vi "main.vi"() -> ()   [LabVIEW 2020]
uses:
  Controls/UI_Cluster.ctl
panel:
  out "I całkujacy":dbl
  out "e uchyb":dbl
  out "c [%] z regulatora":dbl
  in  "Twy [°C] zadane":dbl
  out "Regulator PI":bool
  in  "Dt [s]":dbl=0.2 min=0.2 max=5.0 step=0.1
  out "Wszystko manualnie":bool
  out "Dane wejściowe z pliku":bool
  out "c [%] Moc grzałki z pliku":dbl
  out "Twe [°C] z pliku":dbl
  out "F [L/min] z pliku":dbl
  in  "Radio Buttons":T1(radio)
  in  "Cancel Button":bool
  out "String":string
  in  "Start":bool
  out "Wykres Twy":dbl(graph)
  in  "V [L]":dbl min=0.0
  in  "Prędkość symulacji x":u32(slide) scale=1.0..100.0
  out "Twy [°C]":dbl
  in  "c [%]":dbl min=0.0 max=100.0
  in  "F [L/min]":dbl=5.0 min=0.0
  in  "Twe [°C]":dbl=30.0
  in  "stop":bool
  # "--------------------Dane podane manulanie---------------------"
  # "-----------Dane z pliku-----------"
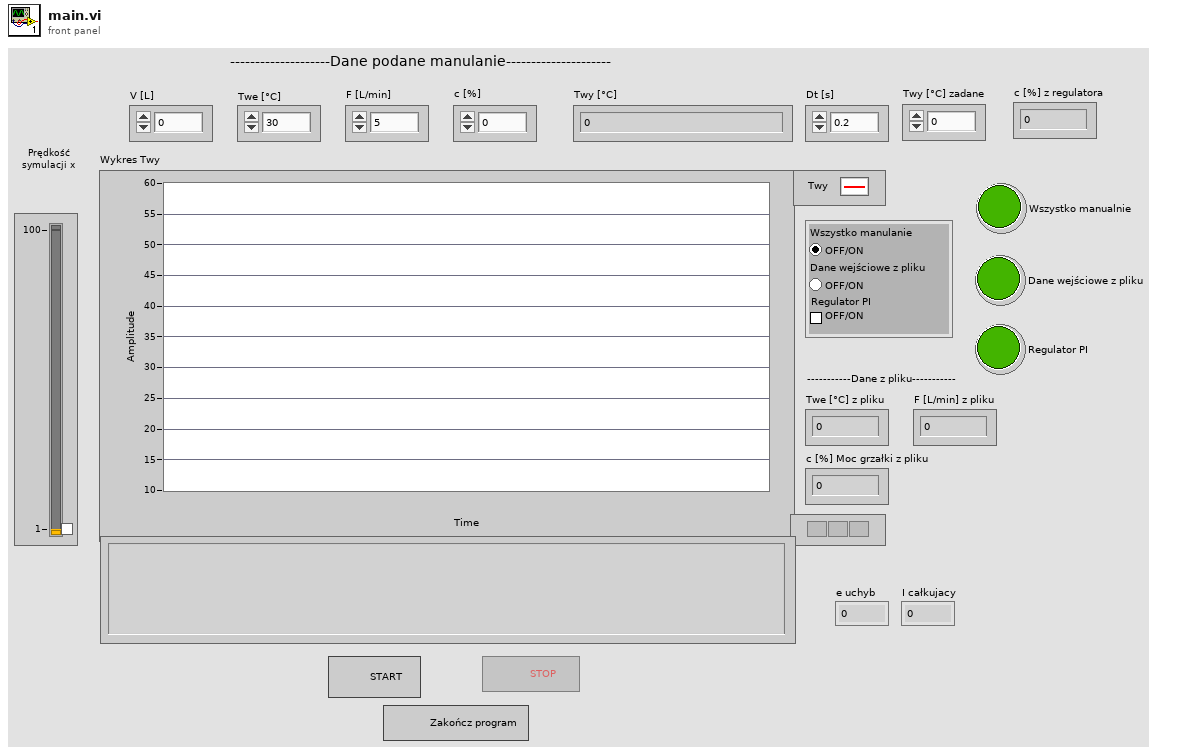
[diagram p1: front panel]
types:
  T1 = enum32{"Wszystko manulanie", "Dane wejściowe z pliku", "Regulator PI"}
  T2 = enum32{"Invalid", "Standard", "Closed", "Hidden", "Minimized", "Maximized"}
  T3 = enum32{"invalid app kind", "Development System", "Run Time System", "Student Edition", "Embedded LabVIEW", "Evaluation", "Custom"}
  T4 = enum16{"open", "replace", "create", "open or create", "replace or create", "replace or create with confirmation"}
  T5 = typedef "UI_Cluster.ctl" = cluster{"krok całkowania Ref":refnum<vi>, "c [%] Ref":refnum<vi>, "F [L/min] Ref":refnum<vi>, "V [L] Ref":refnum<vi>, "Twe Ref":refnum<vi>, "Wykres Twy Ref":refnum<vi>, "String Ref":refnum<vi>, "Start Ref":refnum<vi>, "stop Ref":refnum<vi>, "End Ref":refnum<vi>, "Dane wejściowe z pliku Ref":refnum<vi>, "Wszystko manualnie Ref":refnum<vi>, "Dt Refnum":refnum<vi>, "Radio Buttons Ref":refnum<vi>}
  T6 = cluster{"Core":cluster{"Current VI Reference":refnum<vi>, "Close Panel on Exit?":bool}, "Cluster_OUT":T5}
  T7 = cluster{"Current VI Reference":refnum<vi>, "Close Panel on Exit?":bool}
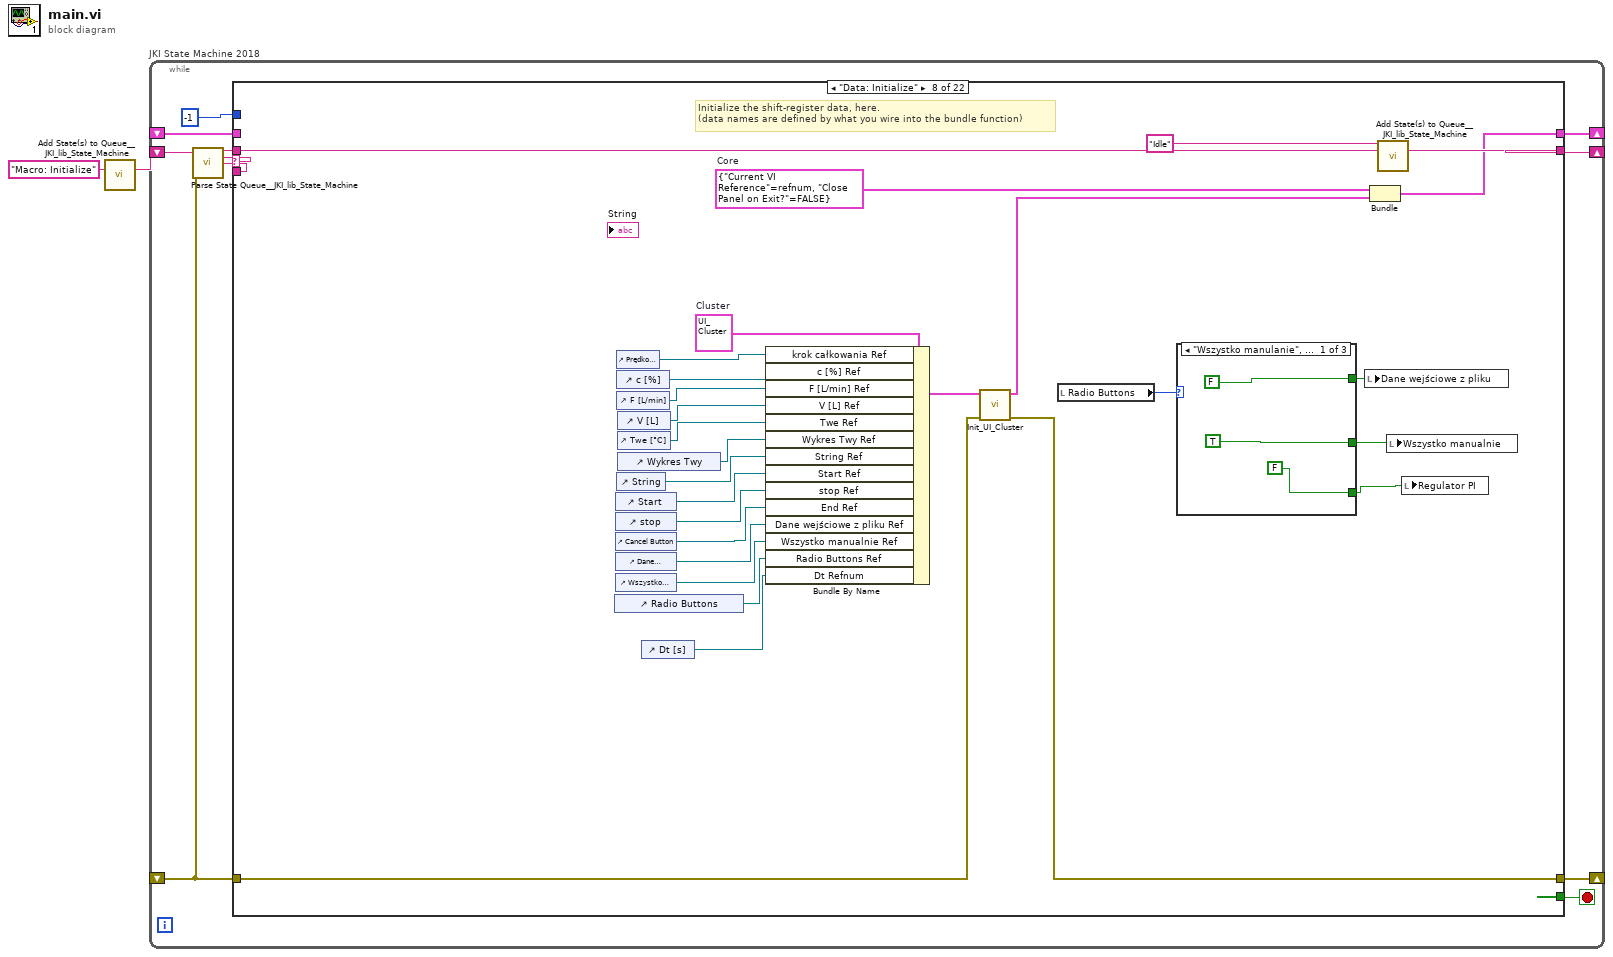
[diagram p0: block diagram]
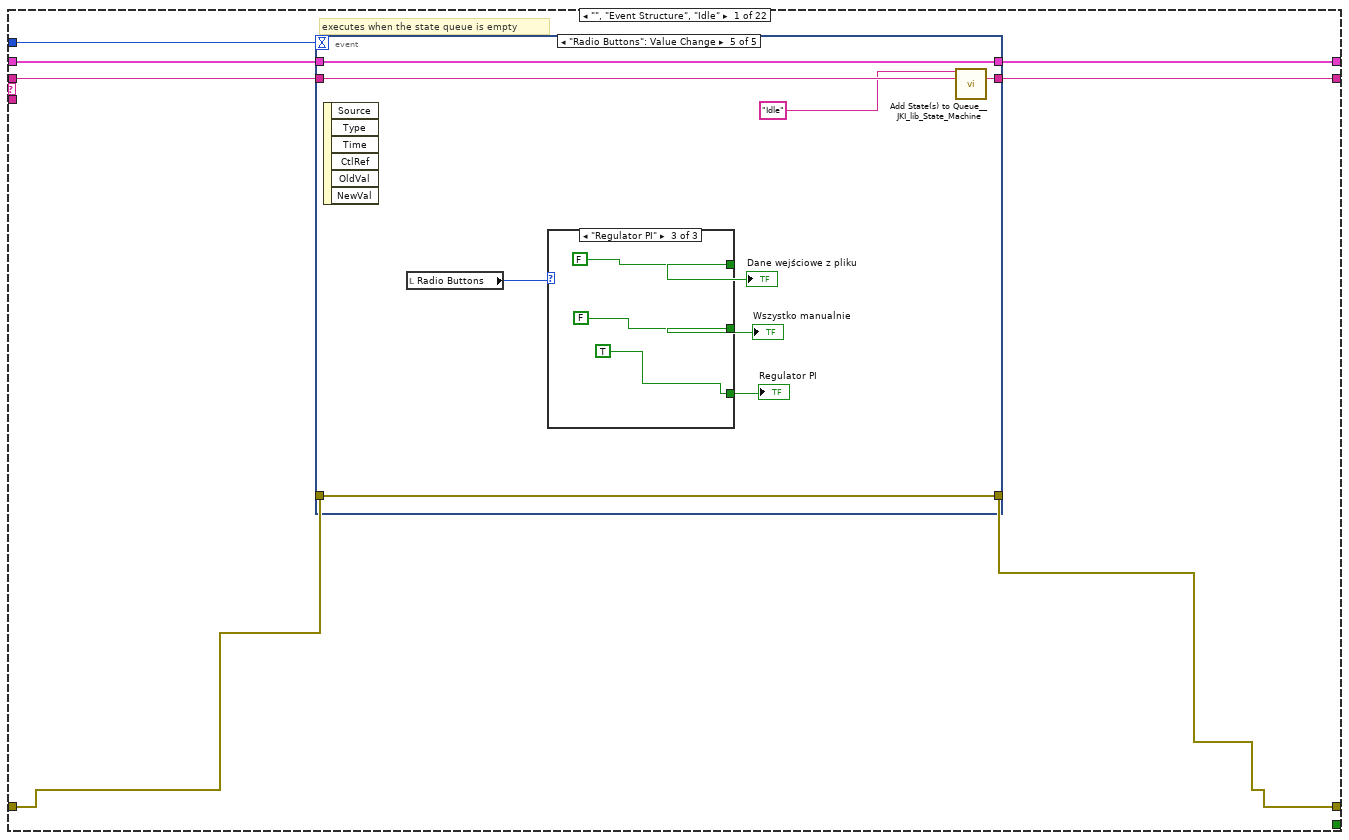
[diagram p2: hidden frame]
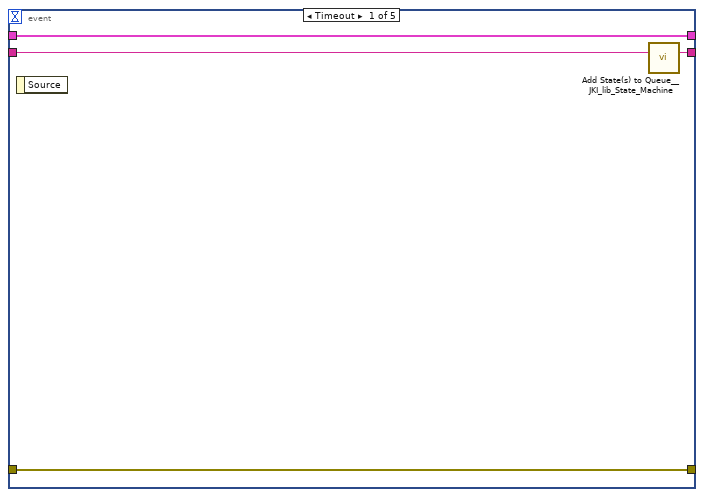
[diagram p3: hidden frame]
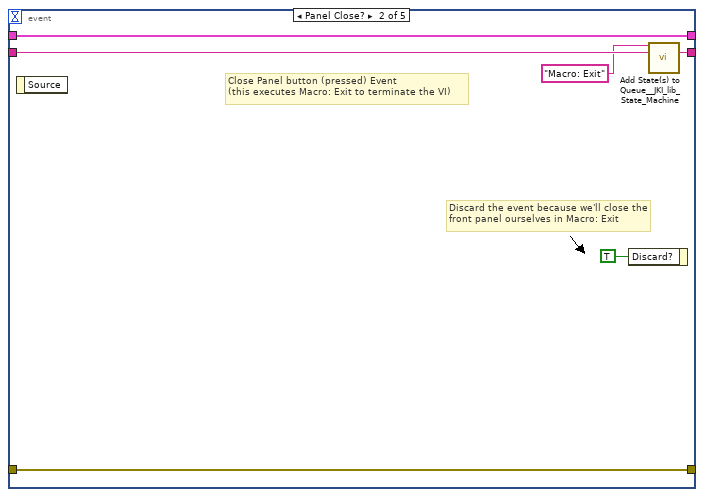
[diagram p4: hidden frame]
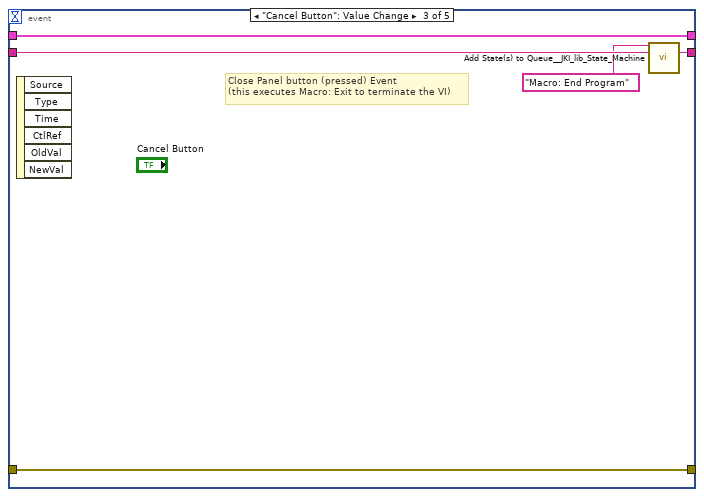
[diagram p5: hidden frame]
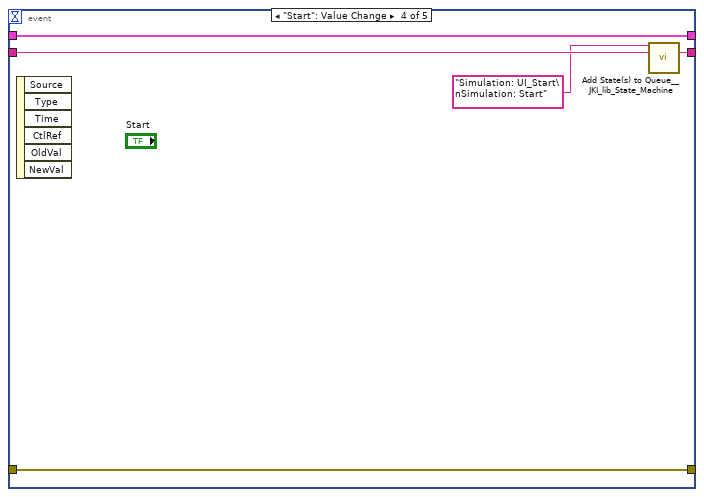
[diagram p6: hidden frame]
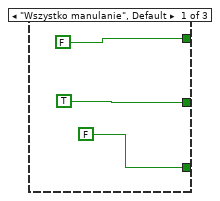
[diagram p7: hidden frame]
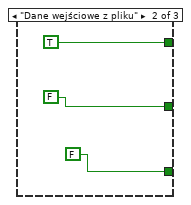
[diagram p8: hidden frame]
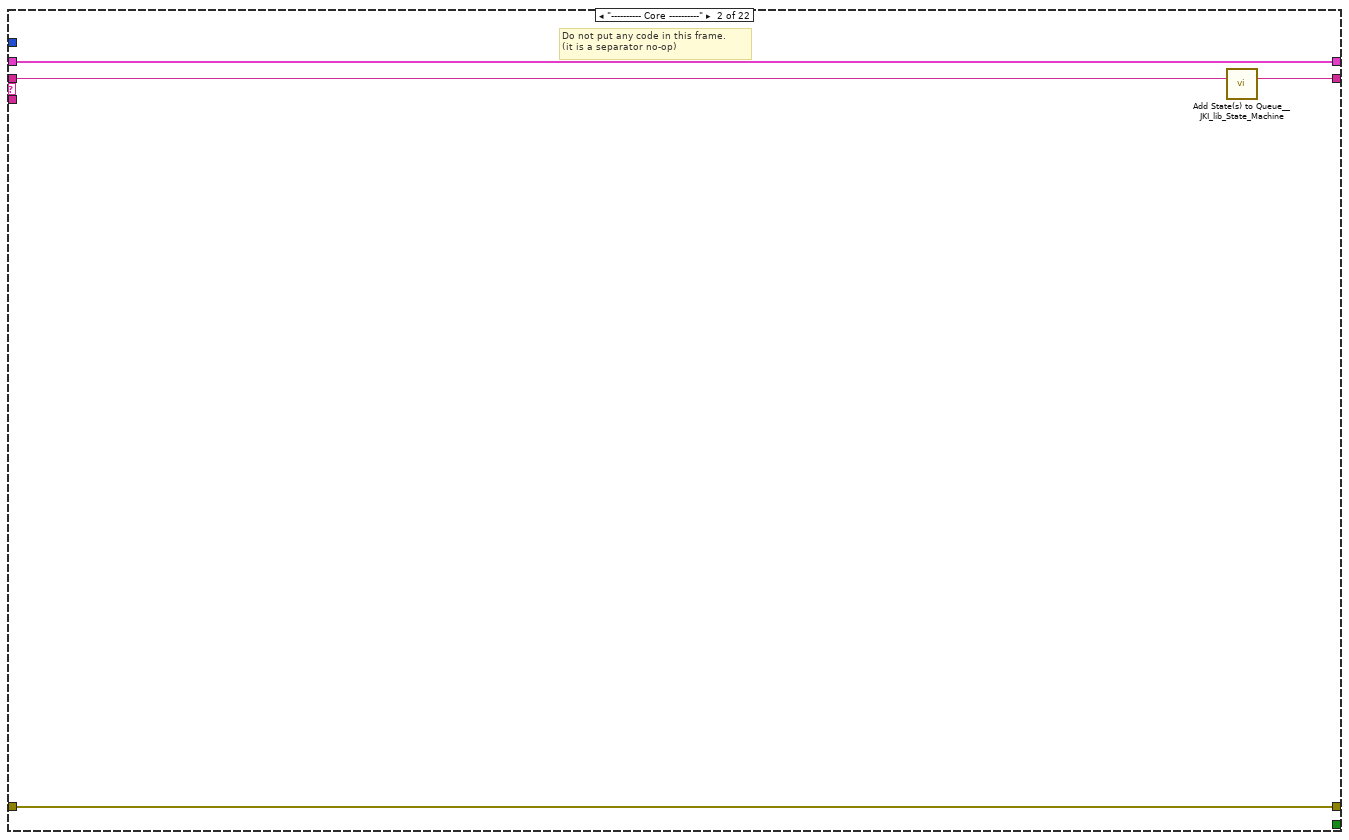
[diagram p9: hidden frame]
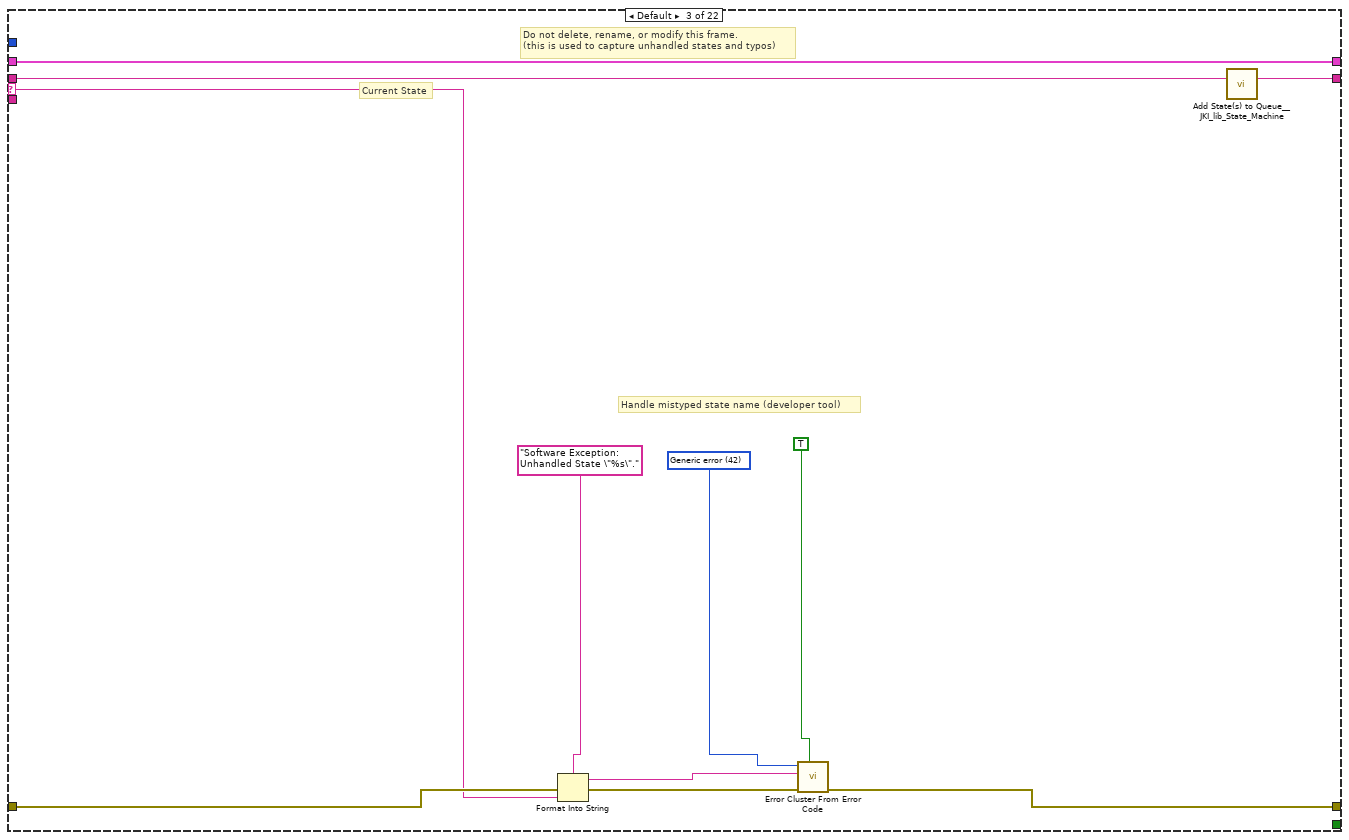
[diagram p10: hidden frame]
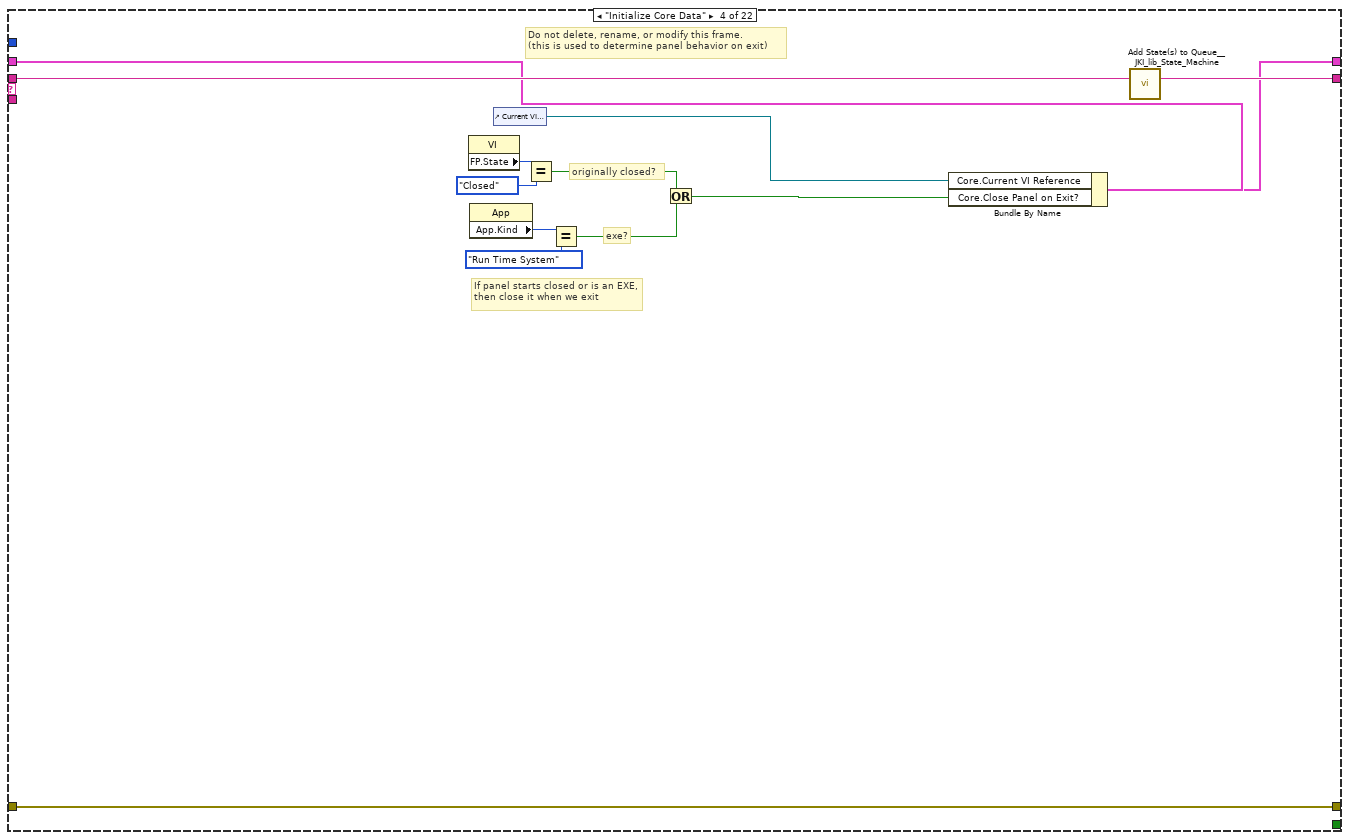
[diagram p11: hidden frame]
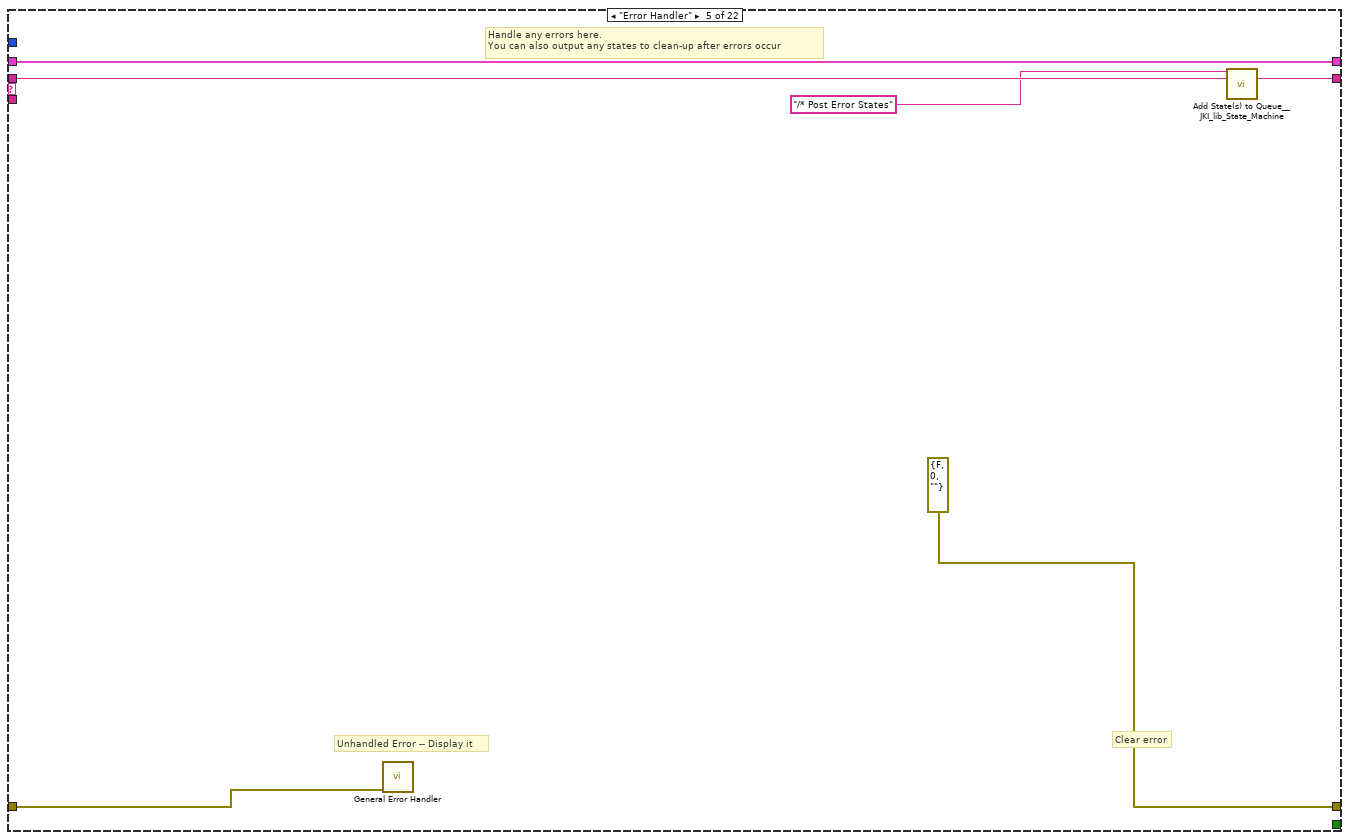
[diagram p12: hidden frame]
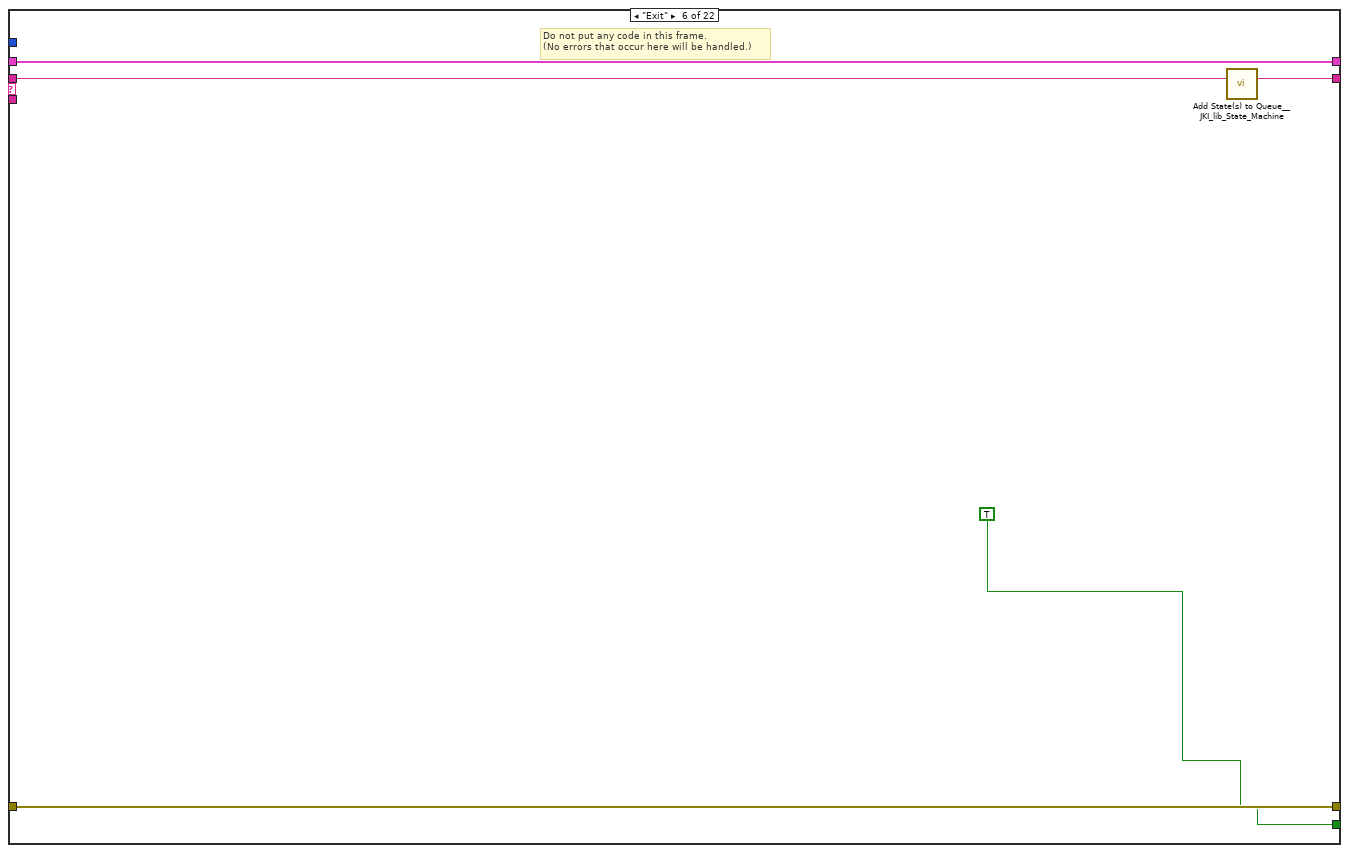
[diagram p13: hidden frame]
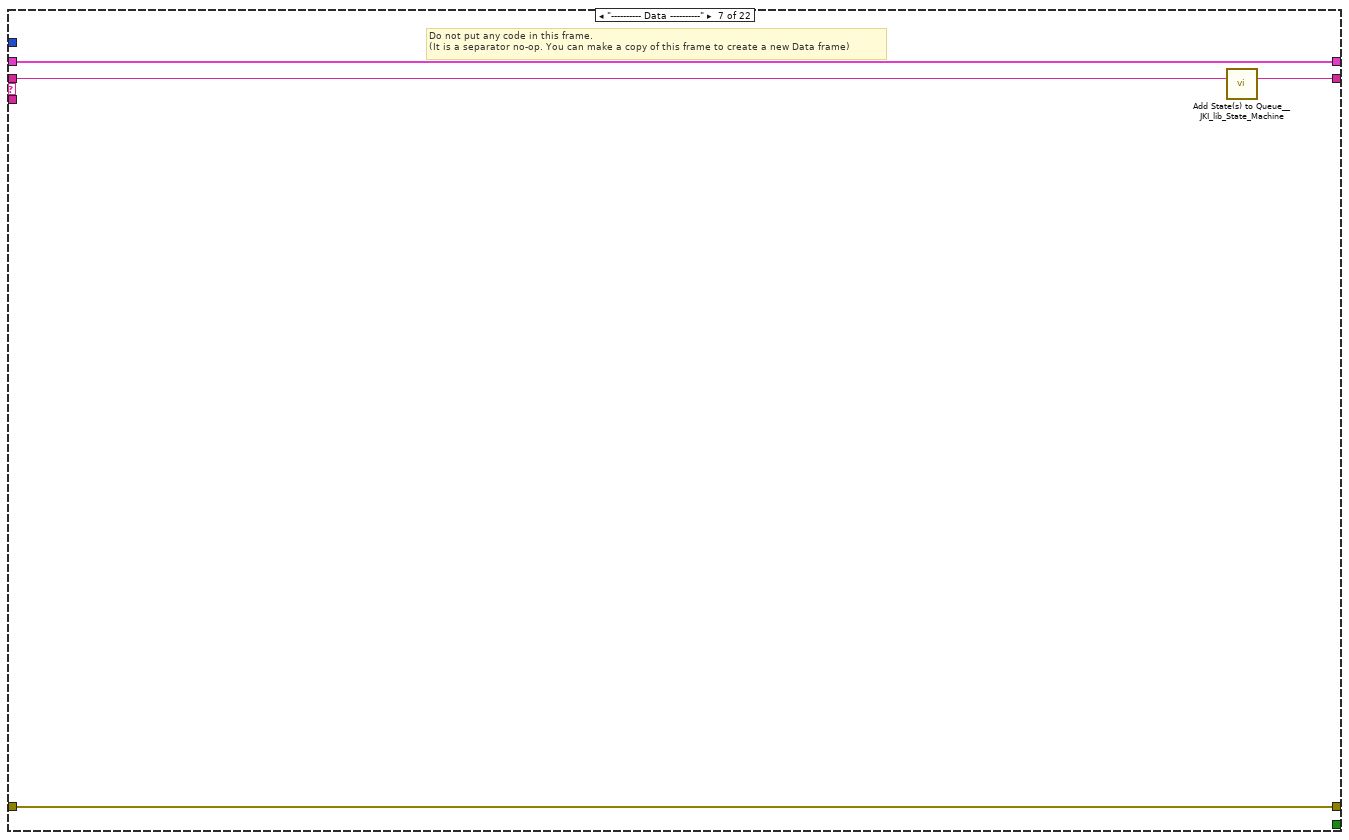
[diagram p14: hidden frame]
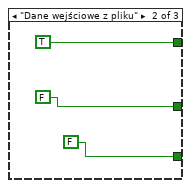
[diagram p15: hidden frame]
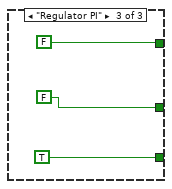
[diagram p16: hidden frame]
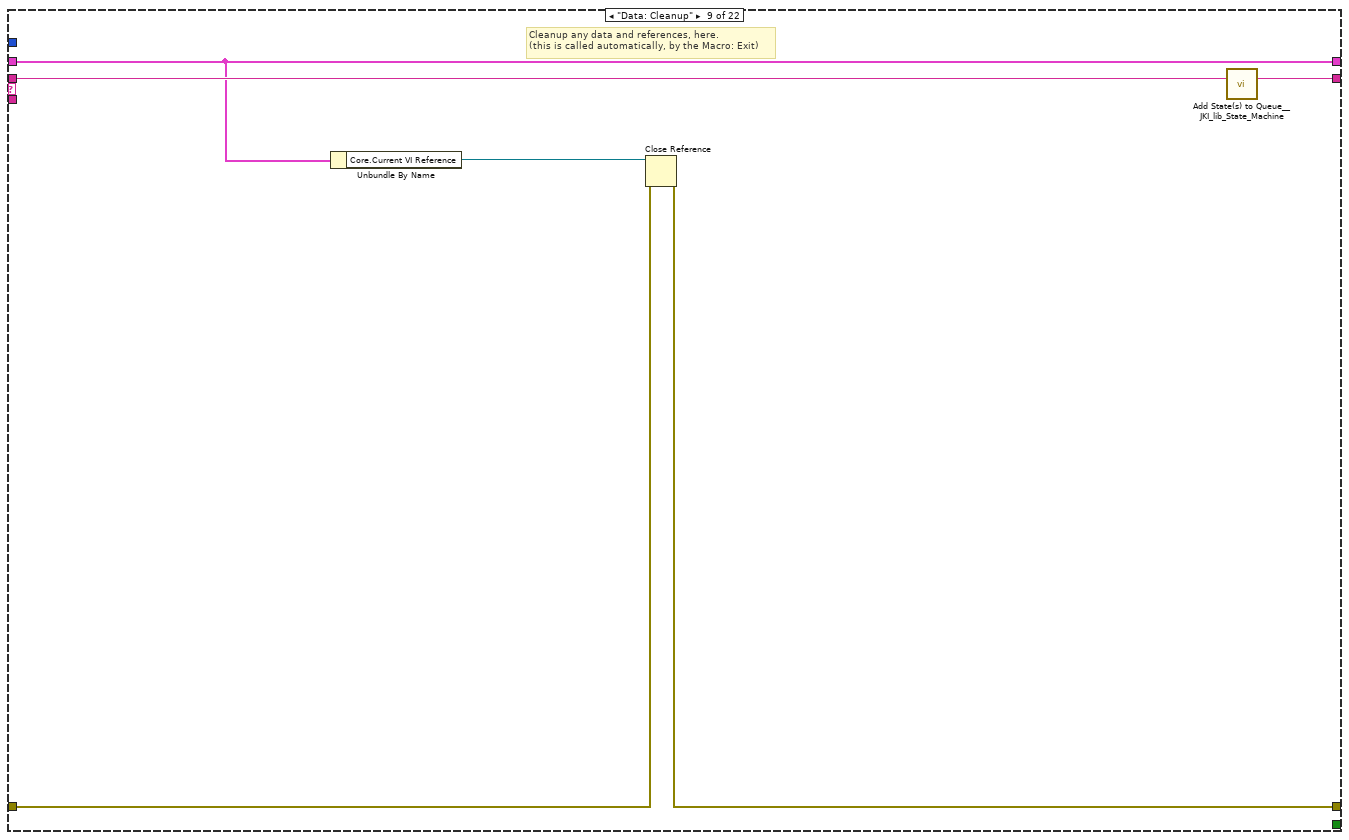
[diagram p17: hidden frame]
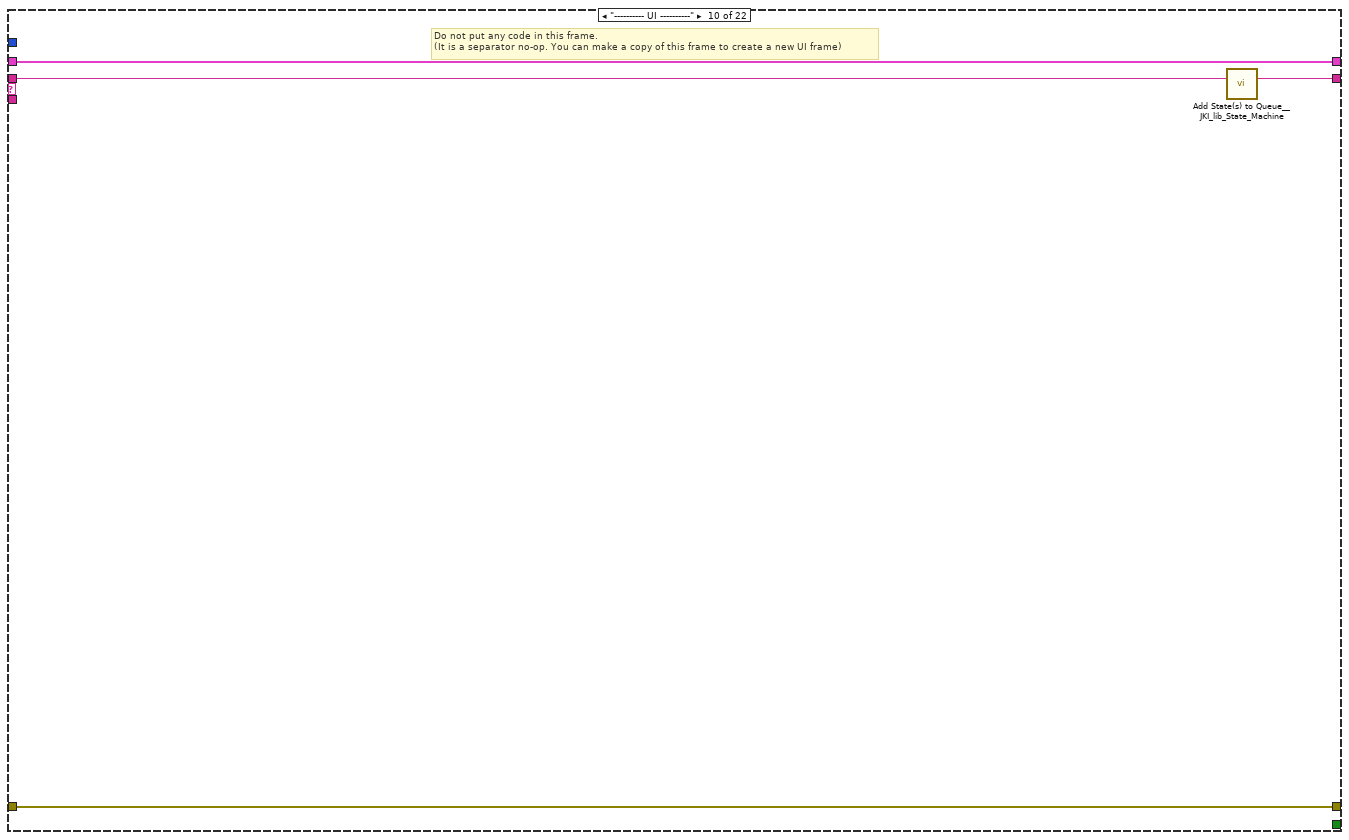
[diagram p18: hidden frame]
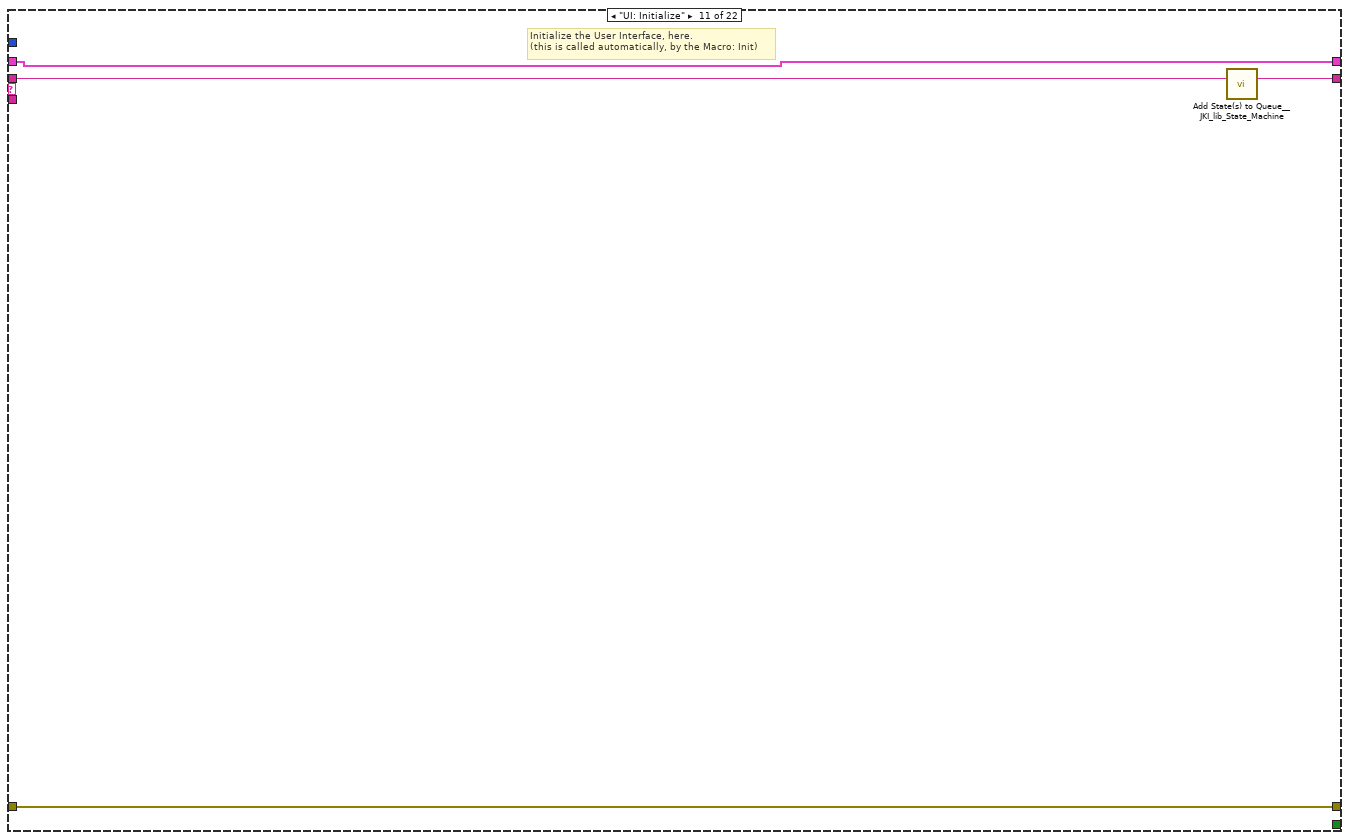
[diagram p19: hidden frame]
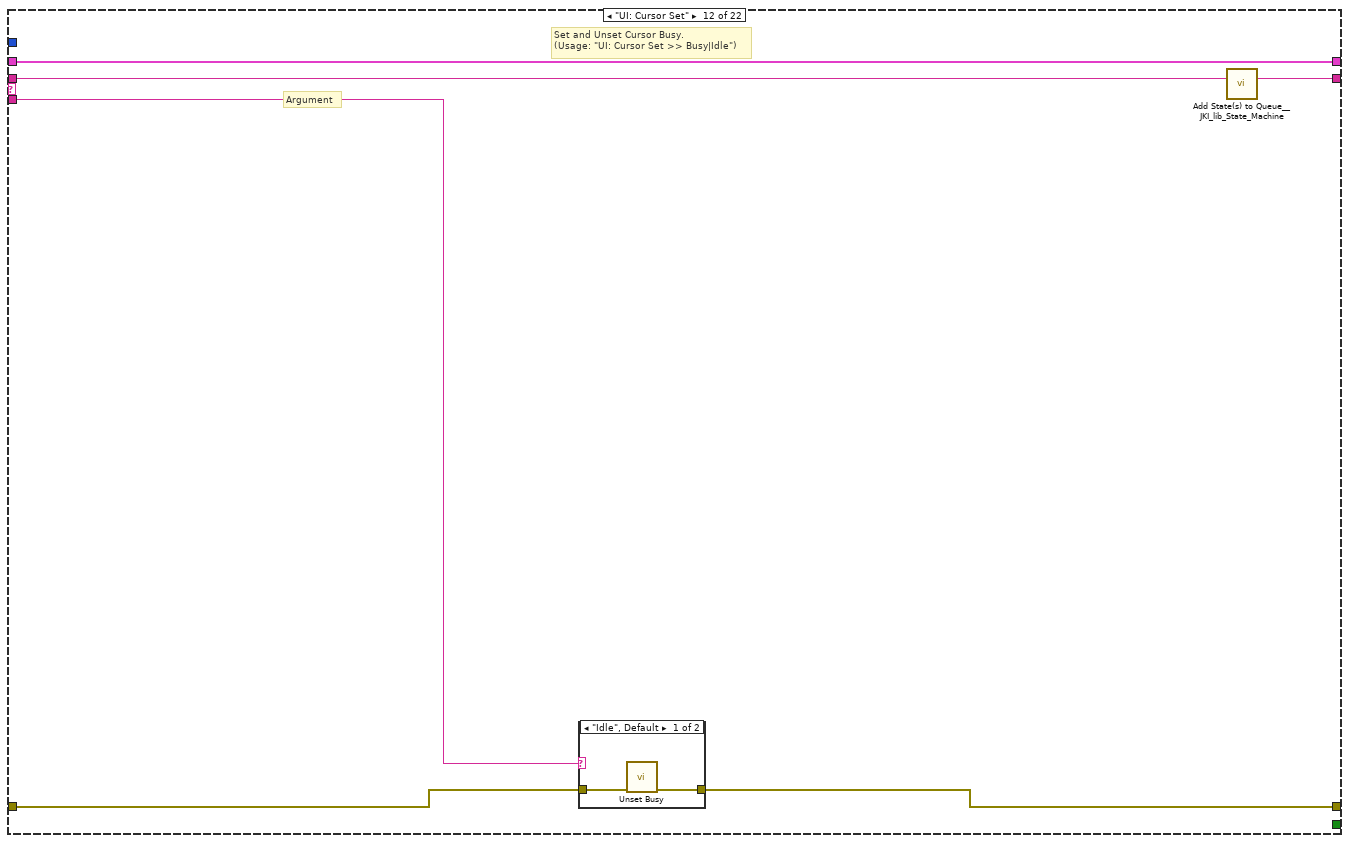
[diagram p20: hidden frame]
diagram:
  n1 = call <vilib>:"Add State(s) to Queue__JKI_lib_State_Machine.vi"("State(s) in (\"\")"="Macro: Initialize") -> ("States Out"=w2:string)  [unwired: 14 in]
  n2 = while "JKI State Machine 2018" {
    shift-right: [w6] -> _
    shift-left: _ -> [w5]
    shift-right: [w9] -> _
    shift-left: _ -> [w3]
    shift-right: [w8] -> _
    shift-left: w2 -> [w10]
    stop <- w7 stop-if-true
    n3 = call <vilib>:"Parse State Queue__JKI_lib_State_Machine.vi"("State Queue"=w10, "Error In (no error)"=w3) -> ("Remaining States"=w12:string, "Current State"=w13:string, "Arguments"=w11:string)  [unwired: 11 in]
    n4 = case shown="\"Data: Initialize\"" w13 {
      selector: w13 -> [_ _ w63 _ _ _ _ _ _ _ _ _ _ _ _ _ _ _ _ _ _ _]
      tunnel: w12 -> [w20 w62 w67 w86 w92 w97 w101 w129 w144 w148 w152 w158 w169 w234 w239 w249 w259 w263 w272 w282 w311 w393]
      tunnel: w11 -> [_ _ _ _ _ _ _ _ _ _ _ w153 w164 _ _ _ _ _ _ _ _ _]
      tunnel: w5 -> [w18 w59 w65 w75 w89 w95 w98 _ w140 w145 w150 w156 w163 w231 w236 w241 w256 w260 w270 w280 w308 w390]
      tunnel: [w17 w60 w69 w84 errorcluster {"status"=FALSE, "code"=0, "source"=""} ("error out") w94 w99 w117 w141 w146 w149 w154 w166 w232 w237 w247 w250 w261 w264 w275 w309 w391] -> w9
      tunnel: w3 -> [w16 w60 w68 w84 w88 w94 w99 w118 w142 w146 w149 w155 w167 w232 w237 w247 w252 w261 w265 w274 w309 w391]
      tunnel: [w19 w61 w66 w85 w91 w96 w100 w128 w143 w147 w151 w157 w168 w233 w238 w248 w258 w262 w271 w281 w310 w392] -> w8
      tunnel: [_ _ _ _ _ TRUE _ _ _ _ _ _ _ _ _ _ TRUE _ _ _ _ _] -> w7
      tunnel: [w15 w59 w65 w74 w89 w95 w98 w115 w140 w145 w150 w156 w163 w231 w236 w241 w256 w260 w266 w278 w308 w390] -> w6
      tunnel: -1 ("Timeout") -> [w14 _ _ _ _ _ _ _ _ _ _ _ _ _ _ _ _ _ _ _ _ _]
      frame "", "Event Structure", "Idle" {
        # "executes when the state queue is empty"
        n5 = event shown="[4] \"Radio Buttons\": Value Change" {
          selector: _ -> [_ _ _ _ _]
          dyn-events: _ -> [_ _ _ _ _]
          timeout: w14 -> [_ _ _ _ _]
          tunnel: w20 -> [w24 w30 w35 w40 w49]
          tunnel: [w23 w29 w34 w39 w48] -> w19
          tunnel: w18 -> [w21 w27 w32 w37 w46]
          tunnel: [w22 w28 w33 w38 w47] -> w17
          tunnel: w16 -> [w22 w28 w33 w38 w47]
          tunnel: [w21 w27 w32 w37 w46] -> w15
          event Timeout {
            n6 = event-data() -> ()  [unwired: 1 in, 1 out]
            n7 = call <vilib>:"Add State(s) to Queue__JKI_lib_State_Machine.vi"("State(s) in (\"\")"=w24) -> ("States Out"=w23:string)  [unwired: 14 in]
          }
          event Panel Close? {
            # "Discard the event because we'll close the front panel ourselves in Macro: Exit"
            # "Close Panel button (pressed) Event\n(this executes Macro: Exit to terminate the VI)"
            n8 = event-data() -> ()  [unwired: 1 in, 1 out]
            n9 = event-data("Discard?"=TRUE) -> ()  [unwired: 1 in, 1 out]
            n10 = call <vilib>:"Add State(s) to Queue__JKI_lib_State_Machine.vi"("State(s) in Front (\"\")"="Macro: Exit", "State(s) in (\"\")"=w30) -> ("States Out"=w29:string)  [unwired: 13 in]
          }
          event "Cancel Button": Value Change {
            # "Close Panel button (pressed) Event\n(this executes Macro: Exit to terminate the VI)"
            n11 = event-data() -> ()  [unwired: 1 in, 6 out]
            n12 = call <vilib>:"Add State(s) to Queue__JKI_lib_State_Machine.vi"("State(s) in Front (\"\")"="Macro: End Program", "State(s) in (\"\")"=w35) -> ("States Out"=w34:string)  [unwired: 13 in]
          }
          event "Start": Value Change {
            n13 = event-data() -> ()  [unwired: 1 in, 6 out]
            n14 = call <vilib>:"Add State(s) to Queue__JKI_lib_State_Machine.vi"("State(s) in Front (\"\")"="Simulation: UI_Start\nSimulation: Start", "State(s) in (\"\")"=w40) -> ("States Out"=w39:string)  [unwired: 13 in]
          }
          event "Radio Buttons": Value Change {
            n15 = event-data() -> ()  [unwired: 1 in, 6 out]
            n16 = local read "Radio Buttons"() -> (w42:T1)
            n17 = case shown="\"Regulator PI\"" w42 {
              tunnel: [FALSE TRUE FALSE] -> w43
              tunnel: [TRUE FALSE FALSE] -> w44
              tunnel: [FALSE FALSE TRUE] -> w41
              frame "Wszystko manulanie", Default {
              }
              frame "Dane wejściowe z pliku" {
              }
              frame "Regulator PI" {
              }
            }
            "Dane wejściowe z pliku" <- w43
            "Wszystko manualnie" <- w44
            "Regulator PI" <- w41
            n18 = call <vilib>:"Add State(s) to Queue__JKI_lib_State_Machine.vi"("State(s) in Front (\"\")"="Idle", "State(s) in (\"\")"=w49) -> ("States Out"=w48:string)  [unwired: 13 in]
          }
        }
      }
      frame "---------- Core ----------" {
        # "Do not put any code in this frame.\n(it is a separator no-op)"
        n19 = call <vilib>:"Add State(s) to Queue__JKI_lib_State_Machine.vi"("State(s) in (\"\")"=w62) -> ("States Out"=w61:string)  [unwired: 14 in]
      }
      frame Default {
        w72 = 42 items=["No error", "Argument error", "Memory is full", "Out of zone", "End of file", "File already open", "Generic file I/O error", "File not found", "File permission error", "Disk is full", "Duplicate path", "Too many files open", "System feature not enabled", "Resource file not found", "Cannot add resource", "Resource not found", "Image not found", "Image memory error", "Pen does not exist", "Config type invalid", "Config token not found", "Config parse error", "Config memory error", "Bad external code format", "Bad external code offset", "External code not present", "Null window", "Destroy window error", "Null menu", "Print aborted", "Bad print record", "Print driver error", "Windows error during printing", "Memory error during printing", "Print dialog error", "Generic print error", "Invalid device refnum", "Device not found", "Device parameter error", "Device unit error", "Cannot open device", "Device call aborted", "Generic error", "Cancelled by user", "Object ID too low", "Object ID too high", "Object not in heap", "Unknown heap", "Unknown object (invalid DefProc)", "Unknown object (DefProc not in table)", "Message out of range", "Invalid (null) method", "Unknown message", "Manager call not supported", "Bad address", "Network operation in progress", "Network operation timed out", "Connection is busy", "Network attribute not supported", "Network error", "Address in use", "System out of memory", "Connection aborted", "Connection refused", "Not connected", "Already connected", "Connection closed", "Initialization error (interapplication manager)", "Bad occurrence", "Wait on unbound occurrence handler", "Occurrence queue overflow", "Datalog type conflict", "Unused", "Unrecognized type (interapplication manager)", "Memory corrupt", "Failed to make temporary DLL", "Old CIN version", "Drag socket not found", "Failed to load drop-object", "Failed to register OLE object", "Failed to release OLE object", "Format specifier type mismatch", "Unknown format specifier", "Too few format specifiers", "Too many format specifiers", "Scan failed", "Newer CIN version", "Error converting to variant", "Runtime menu error", "Password tampered", "Variant attribute not found", "Incompatible variant data type", "Event data is not available", "Event Store is not present", "Occurrence is not found", "Event Queue is not created", "Event info is not available", "Refnum passed is NULL", "Error retrieving Class GUID", "Error retrieving CoClass GUID", "Error retrieving TypeLib GUID.", "Bad built application magic bytes.", "Specific driver is different from the specific driver associated with the Logical Name.", "There is no session opened to the class driver.", "Max Error", "MAX - Error with config objects", "MAX - Error loading configuration", "MAX - Group not supported"]
        # "Current State"
        # "Do not delete, rename, or modify this frame.\n(this is used to capture unhandled states and typos)"
        # "Handle mistyped state name (developer tool)"
        n20 = Format Into String(format string="Software Exception: Unhandled State \"%s\"." ("message"), error in=w68, w63) -> (resulting string=w71:string, error out=w70:errorcluster)  [unwired: 1 in]
        n21 = call <vilib>:"Error Cluster From Error Code.vi"("show call chain? (False)"=TRUE, "error in (no error)"=w70, "error message (\"\")"=w71, "error code (0)"=w72) -> ("error out"=w69:errorcluster)  [unwired: 5 in]
        n22 = call <vilib>:"Add State(s) to Queue__JKI_lib_State_Machine.vi"("State(s) in (\"\")"=w67) -> ("States Out"=w66:string)  [unwired: 14 in]
      }
      frame "Initialize Core Data" {
        # "Do not delete, rename, or modify this frame.\n(this is used to determine panel behavior on exit)"
        # "originally closed?"
        # "exe?"
        # "If panel starts closed or is an EXE, then close it when we exit"
        n23 = property class="VI"() -> ("FP.State"=w78:T2)  [unwired: 2 in, 2 out]
        n24 = property class="App"() -> ("App.Kind"=w83:T3)  [unwired: 2 in, 2 out]
        n25 = control-ref of="Current VI Reference"() -> (w79:refnum<vi>)
        n26 = Equal?(x=w78, y=T2."Closed" ("Front Panel Window:State")) -> (x = y?=w76:bool)
        n27 = Equal?(x=w83, y=T3."Run Time System" ("Application:Kind")) -> (x = y?=w81:bool)
        n28 = Or(x=w76, y=w81) -> (x .or. y?=w80:bool)
        n29 = Bundle By Name(cluster=w75, "Core.Current VI Reference"=w79, "Core.Close Panel on Exit?"=w80) -> (w74:T6)
        n30 = call <vilib>:"Add State(s) to Queue__JKI_lib_State_Machine.vi"("State(s) in (\"\")"=w86) -> ("States Out"=w85:string)  [unwired: 14 in]
      }
      frame "Error Handler" {
        # "Unhandled Error -- Display it"
        # "Handle any errors here.\nYou can also output any states to clean-up after errors occur"
        # "Clear error"
        n31 = call <vilib>:"General Error Handler.vi"("error in (no error)"=w88) -> ()  [unwired: 10 in, 5 out]
        n32 = call <vilib>:"Add State(s) to Queue__JKI_lib_State_Machine.vi"("State(s) in Front (\"\")"="/* Post Error States", "State(s) in (\"\")"=w92) -> ("States Out"=w91:string)  [unwired: 13 in]
      }
      frame "Exit" {
        # "Do not put any code in this frame.\n(No errors that occur here will be handled.)"
        n33 = call <vilib>:"Add State(s) to Queue__JKI_lib_State_Machine.vi"("State(s) in (\"\")"=w97) -> ("States Out"=w96:string)  [unwired: 14 in]
      }
      frame "---------- Data ----------" {
        # "Do not put any code in this frame.\n(It is a separator no-op. You can make a copy of this frame to create a new Data frame)"
        n34 = call <vilib>:"Add State(s) to Queue__JKI_lib_State_Machine.vi"("State(s) in (\"\")"=w101) -> ("States Out"=w100:string)  [unwired: 14 in]
      }
      frame "Data: Initialize" {
        w120 = T5 {"krok całkowania Ref"=refnum, "c [%] Ref"=refnum, "F [L/min] Ref"=refnum, "V [L] Ref"=refnum, "Twe Ref"=refnum, "Wykres Twy Ref"=refnum, "String Ref"=refnum, "Start Ref"=refnum, "stop Ref"=refnum, "End Ref"=refnum, "Dane wejściowe z pliku Ref"=refnum, "Wszystko manualnie Ref"=refnum, "Dt Refnum"=refnum, "Radio Buttons Ref"=refnum}  # Cluster
        w127 = T7 {"Current VI Reference"=refnum, "Close Panel on Exit?"=FALSE}  # Core
        # "Initialize the shift-register data, here.\n(data names are defined by what you wire into the bundle function)"
        n35 = control-ref of="Radio Buttons"() -> (w107:refnum<vi>)
        n36 = control-ref of="Start"() -> (w112:refnum<vi>)
        n37 = control-ref of="stop"() -> (w111:refnum<vi>)
        n38 = control-ref of="Cancel Button"() -> (w110:refnum<vi>)
        n39 = control-ref of="Dane wejściowe z pliku"() -> (w109:refnum<vi>)
        n40 = control-ref of="Wszystko manualnie"() -> (w108:refnum<vi>)
        n41 = control-ref of="Prędkość symulacji x"() -> (w126:refnum<vi>)
        n42 = control-ref of="c [%]"() -> (w125:refnum<vi>)
        n43 = control-ref of="F [L/min]"() -> (w124:refnum<vi>)
        n44 = control-ref of="String"() -> (w114:refnum<vi>)
        n45 = control-ref of="V [L]"() -> (w123:refnum<vi>)
        n46 = control-ref of="Twe [°C]"() -> (w122:refnum<vi>)
        n47 = control-ref of="Wykres Twy"() -> (w121:refnum<vi>)
        n48 = control-ref of="Dt [s]"() -> (w103:refnum<vi>)
        n49 = Bundle By Name(cluster=w120, "krok całkowania Ref"=w126, "c [%] Ref"=w125, "F [L/min] Ref"=w124, "V [L] Ref"=w123, "Twe Ref"=w122, "Wykres Twy Ref"=w121, "String Ref"=w114, "Start Ref"=w112, "stop Ref"=w111, "End Ref"=w110, "Dane wejściowe z pliku Ref"=w109, "Wszystko manualnie Ref"=w108, "Radio Buttons Ref"=w107, "Dt Refnum"=w103) -> (w119:T5)
        n50 = call "Init_UI_Cluster.vi"("error in (no error)"=w118, "Cluster_IN"=w119) -> ("error out"=w117:errorcluster, "Cluster_OUT"=w116:T5)  [unwired: 8 in]
        n51 = local read "Radio Buttons"() -> (w106:T1)
        n52 = case shown="\"Wszystko manulanie\", Default" w106 {
          tunnel: [FALSE TRUE FALSE] -> w105
          tunnel: [TRUE FALSE FALSE] -> w104
          tunnel: [FALSE FALSE TRUE] -> w102
          frame "Wszystko manulanie", Default {
          }
          frame "Dane wejściowe z pliku" {
          }
          frame "Regulator PI" {
          }
        }
        n53 = local write "Dane wejściowe z pliku"(w105) -> ()
        n54 = Bundle("Core"=w127, "Cluster_OUT"=w116) -> (w115:T6)  [unwired: 1 in]
        n55 = call <vilib>:"Add State(s) to Queue__JKI_lib_State_Machine.vi"("State(s) in Front (\"\")"="Idle" ("State(s) in Front (\"\")"), "State(s) in (\"\")"=w129) -> ("States Out"=w128:string)  [unwired: 13 in]
        n56 = local write "Wszystko manualnie"(w104) -> ()
        n57 = local write "Regulator PI"(w102) -> ()
      }
      frame "Data: Cleanup" {
        # "Cleanup any data and references, here.\n(this is called automatically, by the Macro: Exit)"
        n58 = Unbundle By Name(w140) -> ("Core.Current VI Reference"=w139:refnum<vi>)
        n59 = Close Reference(reference=w139, error in (no error)=w142) -> (error out=w141:errorcluster)
        n60 = call <vilib>:"Add State(s) to Queue__JKI_lib_State_Machine.vi"("State(s) in (\"\")"=w144) -> ("States Out"=w143:string)  [unwired: 14 in]
      }
      frame "---------- UI ----------" {
        # "Do not put any code in this frame.\n(It is a separator no-op. You can make a copy of this frame to create a new UI frame)"
        n61 = call <vilib>:"Add State(s) to Queue__JKI_lib_State_Machine.vi"("State(s) in (\"\")"=w148) -> ("States Out"=w147:string)  [unwired: 14 in]
      }
      frame "UI: Initialize" {
        # "Initialize the User Interface, here.\n(this is called automatically, by the Macro: Init)"
        n62 = call <vilib>:"Add State(s) to Queue__JKI_lib_State_Machine.vi"("State(s) in (\"\")"=w152) -> ("States Out"=w151:string)  [unwired: 14 in]
      }
      frame "UI: Cursor Set" {
        # "Argument"
        # "Set and Unset Cursor Busy.\n(Usage: \"UI: Cursor Set >> Busy|Idle\")"
        n63 = case shown="\"Idle\", Default" w153 {
          tunnel: w155 -> [w160 w162]
          tunnel: [w159 w161] -> w154
          frame "Idle", Default {
            n64 = call <vilib>:"Unset Busy.vi"("error in (no error)"=w160) -> ("error out"=w159:errorcluster)  [unwired: 10 in]
          }
          frame "Busy" {
            n65 = call <vilib>:"Set Busy.vi"("error in (no error)"=w162) -> ("error out"=w161:errorcluster)  [unwired: 9 in, 1 out]
          }
        }
        n66 = call <vilib>:"Add State(s) to Queue__JKI_lib_State_Machine.vi"("State(s) in (\"\")"=w158) -> ("States Out"=w157:string)  [unwired: 14 in]
      }
      frame "UI: Front Panel State" {
        # "Argument"
        # "Set Front Panel Open or Closed\n(Usage: \"UI: Front Panel State >> Open|Close\")"
        n67 = Unbundle By Name(w163) -> ("Core.Current VI Reference"=w165:refnum<vi>)
        n68 = case shown="\"Minimize\", \"Minimized\"" w164 {
          tunnel: w167 -> [w175 w188 w199 w212 w224]
          tunnel: [w176 w189 w200 w213 w225] -> w166
          tunnel: w165 -> [_ _ _ w206 _]
          frame "Open", "Standard", Default {
            w170 = T2."Standard" ("State")
            n69 = property class="VI"(error in=w175) -> (reference out=w173:refnum<vi>, error out=w174:errorcluster, "FP.State"=w172:T2)  [unwired: 1 in]
            n70 = Not Equal?(x=w172, y=w170) -> (x != y?=w171:bool)
            n71 = case shown="True" w171 {
              tunnel: [w180 w182] -> w176
              tunnel: w174 -> [w179 w182]
              tunnel: w173 -> [w178 _]
              tunnel: w170 -> [w177 _]
              frame True {
                n72 = invoke class="VI" method="FP.Open"(reference=w178, error in=w179, "Activate"=TRUE, "State"=w177) -> (error out=w180:errorcluster)  [unwired: 1 in, 4 out]
              }
              frame False {
              }
            }
          }
          frame "Close", "Closed" {
            n73 = property class="VI"(error in=w188) -> (reference out=w186:refnum<vi>, error out=w187:errorcluster, "FP.State"=w184:T2)  [unwired: 1 in]
            n74 = Not Equal?(x=w184, y=T2."Closed" ("Front Panel Window:State")) -> (x != y?=w183:bool)
            n75 = case shown="True" w183 {
              tunnel: [w190 w193] -> w189
              tunnel: w187 -> [w190 w192]
              tunnel: w186 -> [_ w191]
              frame False {
              }
              frame True {
                n76 = invoke class="VI" method="FP.Close"(reference=w191, error in=w192) -> (error out=w193:errorcluster)  [unwired: 1 in, 2 out]
              }
            }
          }
          frame "Hidden", "Hide" {
            w194 = T2."Hidden" ("State")
            n77 = property class="VI"(error in=w199) -> (reference out=w197:refnum<vi>, error out=w198:errorcluster, "FP.State"=w196:T2)  [unwired: 1 in]
            n78 = Not Equal?(x=w196, y=w194) -> (x != y?=w195:bool)
            n79 = case shown="True" w195 {
              tunnel: [w204 w205] -> w200
              tunnel: w198 -> [w203 w205]
              tunnel: w197 -> [w202 _]
              tunnel: w194 -> [w201 _]
              frame True {
                n80 = invoke class="VI" method="FP.Open"(reference=w202, error in=w203, "State"=w201) -> (error out=w204:errorcluster)  [unwired: 2 in, 4 out]
              }
              frame False {
              }
            }
          }
          frame "Minimize", "Minimized" {
            w207 = T2."Minimized" ("State")
            n81 = property class="VI"(reference=w206, error in=w212) -> (reference out=w210:refnum<vi>, error out=w211:errorcluster, "FP.State"=w209:T2)
            n82 = Not Equal?(x=w209, y=w207) -> (x != y?=w208:bool)
            n83 = case shown="True" w208 {
              tunnel: [w217 w218] -> w213
              tunnel: w211 -> [w216 w218]
              tunnel: w210 -> [w215 _]
              tunnel: w207 -> [w214 _]
              frame True {
                n84 = invoke class="VI" method="FP.Open"(reference=w215, error in=w216, "State"=w214) -> (error out=w217:errorcluster)  [unwired: 2 in, 4 out]
              }
              frame False {
              }
            }
          }
          frame "Maximize", "Maximized" {
            w219 = T2."Maximized" ("State")
            n85 = property class="VI"(error in=w224) -> (reference out=w222:refnum<vi>, error out=w223:errorcluster, "FP.State"=w221:T2)  [unwired: 1 in]
            n86 = Not Equal?(x=w221, y=w219) -> (x != y?=w220:bool)
            n87 = case shown="True" w220 {
              tunnel: [w229 w230] -> w225
              tunnel: w223 -> [w228 w230]
              tunnel: w222 -> [w227 _]
              tunnel: w219 -> [w226 _]
              frame True {
                n88 = invoke class="VI" method="FP.Open"(reference=w227, error in=w228, "State"=w226) -> (error out=w229:errorcluster)  [unwired: 2 in, 4 out]
              }
              frame False {
              }
            }
          }
        }
        n89 = call <vilib>:"Add State(s) to Queue__JKI_lib_State_Machine.vi"("State(s) in (\"\")"=w169) -> ("States Out"=w168:string)  [unwired: 14 in]
      }
      frame "---------- Macro ----------" {
        # "Do not put any code in this frame.\n(It is a separator no-op. You can make a copy of this frame to create a new Macro frame)"
        n90 = call <vilib>:"Add State(s) to Queue__JKI_lib_State_Machine.vi"("State(s) in (\"\")"=w234) -> ("States Out"=w233:string)  [unwired: 14 in]
      }
      frame "Macro: Initialize" {
        w235 = "Data: Initialize\nInitialize Core Data\nUI: Initialize\nUI: Front Panel State >> Open"  # Data: Initialize Initialize Core Data UI: Initialize UI: Front Panel State >> Open
        # "Initialization Macro\n(This is called once, when the VI starts)"
        n91 = call <vilib>:"Add State(s) to Queue__JKI_lib_State_Machine.vi"("State(s) in Front (\"\")"=w235, "State(s) in (\"\")"=w239) -> ("States Out"=w238:string)  [unwired: 13 in]
      }
      frame "Macro: Exit" {
        # "Exit Macro\n(This is called once, when the VI exits)"
        n92 = Unbundle By Name(w241) -> ("Core.Close Panel on Exit?"=w240:bool)
        n93 = Select(t="UI: Front Panel State >> Close", s=w240, f="") -> (s? t:f=w244:string)
        n94 = call <vilib>:"Add State(s) to Queue__JKI_lib_State_Machine.vi"("State(s) in (\"\")"=w244, "State(s) at Back (\"\")"="Data: Cleanup\nExit") -> ("States Out"=w242:string)  [unwired: 13 in]
        n95 = call <vilib>:"Add State(s) to Queue__JKI_lib_State_Machine.vi"("State(s) in Front (\"\")"=w242, "State(s) in (\"\")"=w249) -> ("States Out"=w248:string)  [unwired: 13 in]
      }
      frame "Macro: End Program" {
        # "Exit Macro\n(This is called once, when the VI exits)"
        n96 = Unbundle By Name(w256) -> ("Cluster_OUT.String Ref"=w255:refnum<vi>)
        n97 = property class="Str"(reference=w255, error in=w252, "Value"="Zakończono program.") -> (reference out=w253:refnum<vi>, error out=w251:errorcluster)
        n98 = Close Reference(reference=w253, error in (no error)=w251) -> (error out=w250:errorcluster)
        n99 = call <vilib>:"Add State(s) to Queue__JKI_lib_State_Machine.vi"("State(s) in (\"\")"=w259) -> ("States Out"=w258:string)  [unwired: 14 in]
      }
      frame "---------- Simulation ----------" {
        # "Template Separator\n(You can make a copy of, or modify, this frame)"
        n100 = call <vilib>:"Add State(s) to Queue__JKI_lib_State_Machine.vi"("State(s) in (\"\")"=w263) -> ("States Out"=w262:string)  [unwired: 14 in]
      }
      frame "Simulation: UI_Start" {
        n101 = Unbundle(w270) -> ("Core"=w267:T7, "Cluster_OUT"=w269:T5)
        n102 = call "Init_UI_Start.vi"("error in (no error)"=w265, "Cluster_IN"=w269) -> ("error out"=w264:errorcluster, "Cluster_OUT"=w268:T5)  [unwired: 8 in]
        n103 = Bundle("Core"=w267, "Cluster_OUT"=w268) -> (w266:T6)  [unwired: 1 in]
        n104 = call <vilib>:"Add State(s) to Queue__JKI_lib_State_Machine.vi"("State(s) in (\"\")"=w272) -> ("States Out"=w271:string)  [unwired: 14 in]
      }
      frame "Simulation: UI_Stop" {
        n105 = Unbundle(w280) -> ("Core"=w279:T7, "Cluster_OUT"=w277:T5)
        n106 = call "Init_UI_Stop.vi"("error in (no error)"=w274, "Cluster_IN"=w277) -> ("error out"=w275:errorcluster, "Cluster_OUT"=w276:T5)  [unwired: 8 in]
        n107 = Bundle("Core"=w279, "Cluster_OUT"=w276) -> (w278:T6)  [unwired: 1 in]
        n108 = call <vilib>:"Add State(s) to Queue__JKI_lib_State_Machine.vi"("State(s) in Front (\"\")"="Idle" ("State(s) in Front (\"\")"), "State(s) in (\"\")"=w282) -> ("States Out"=w281:string)  [unwired: 13 in]
      }
      frame "Simulation: Start" {
        # "Your code here.\n(You can make a copy of, or modify, this frame)"
        n109 = local read "Radio Buttons"() -> (w294:T1)
        n110 = call <vilib>:"Application Directory.vi"() -> ("Application Directory"=w286:path)
        n111 = call <vilib>:"Application Directory.vi"() -> ("Application Directory"=w287:path)
        n112 = Build Path(base path=w286, name or relative path=path "Dane_zapis.txt") -> (appended path=w288:path)
        n113 = Build Path(base path=w287, name or relative path=path "chka_F_Pg30.txt") -> (appended path=w290:path)
        n114 = call "Dane_wej.vi"("file path (use dialog)"=w290) -> ("L/min"=w295:dbl, "Twe"=w292:dbl, "Moc grzałki"=w296:dbl)  [unwired: 8 in]
        n115 = case shown="\"Wszystko manulanie\", Default" w294 {
          tunnel: [w312 w313] -> w293
          tunnel: w292 -> [_ w313]
          frame "Wszystko manulanie", Default {
            n116 = local read "Twe [°C]"() -> (w312:dbl)
          }
          frame "Dane wejściowe z pliku" {
          }
        }
        n117 = Open/Create/Replace File(file path (use dialog)=w288, operation (0:open)=T4."open", access (0:read/write)=enum16{"read/write", "read-only", "write-only"}."write-only") -> (refnum out=w300:refnum<file>, error out=w299:errorcluster)  [unwired: 3 in, 1 out]
        n118 = while {
          shift-right: [w335] -> _
          shift-left: w293 -> [w342]
          tunnel: "Twe [°C]" -> [w327]
          tunnel: "c [%]" -> [w325]
          tunnel: "F [L/min]" -> [w326]
          tunnel: "V [L]" -> [w341]
          tunnel: w300 -> [w340]
          tunnel: w299 -> [w339]
          tunnel: [w338] -> w298
          tunnel: [w337] -> w297
          tunnel: w296 -> [w330]
          tunnel: w292 -> [w329]
          tunnel: w295 -> [w328]
          tunnel: "Dt [s]" -> [w322]
          tunnel: "Dt [s]" -> [w320]
          shift-right: [w317] -> _
          shift-left: 0.0 ("I") -> [w316]
          shift-right: [w315] -> _
          shift-left: 0.0 ("c") -> [w314]
          stop <- "stop" stop-if-true
          n119 = Multiply(x=w320, y=1000.0) -> (x*y=w319:dbl)
          n120 = Divide(x=w319, y="Prędkość symulacji x") -> (x/y=w324:dbl)
          n121 = Wait Until Next ms Multiple(millisecond multiple=w324) -> ()  [unwired: 1 out]
          n122 = case shown="\"Regulator PI\"" "Radio Buttons" {
            tunnel: w342 -> [w350 w370 w389]
            tunnel: w341 -> [w349 w369 w380]
            tunnel: [w348 w368 w379] -> w335
            tunnel: w330 -> [_ _ w378]
            tunnel: w329 -> [_ _ w377]
            tunnel: w328 -> [_ _ w376]
            tunnel: w327 -> [w347 w367 _]
            tunnel: w326 -> [w346 w366 _]
            tunnel: w325 -> [w345 _ _]
            tunnel: w322 -> [w344 w365 w375]
            tunnel: [_ w362 _] -> w317
            tunnel: w316 -> [_ w361 _]
            tunnel: [_ w359 _] -> w315
            tunnel: w314 -> [_ w360 _]
            frame "Wszystko manulanie", Default {
              n123 = Divide(x=w345, y=100.0) -> (x/y=w358:dbl)
              n124 = Divide(x=w349, y=1000.0) -> (x/y=w353:dbl)
              n125 = Multiply(x=w358, y=12200.0) -> (x*y=w352:dbl)
              n126 = Divide(x=w346, y=60000.0) -> (x/y=w351:dbl)
              n127 = formula code="float T = V/F;\nfloat ro = 997.3;\nfloat cw = 4200;\n\nint NIS =1000;\nint m;\nfor(m=0 ; m<NIS; m++)\n{\n float h = Dt/NIS;\nfloat G=F/V*(Twe-Twy)+Pc/(ro*cw*V);\nTwy=Twy+G*h;\n}"("Pc"=w352, "F"=w351, "Twe"=w347, "V"=w353, "Twy"=w350, "Dt"=w344) -> ("Twy"=w348:dbl)
            }
            frame "Regulator PI" {
              n128 = Divide(x=w369, y=1000.0) -> (x/y=w372:dbl)
              n129 = Divide(x=w366, y=60000.0) -> (x/y=w371:dbl)
              n130 = formula code="float T = V/F;\nfloat ro = 997.3;\nfloat cw = 4200;\nfloat e; \nint moc_grzalki = 12200;\n float Pc;\nint NIS =1000; int m;\nfloat P; \nfloat Ti = 5; float kp = 20;\n\ne = Twy_zad - Twy;\nP = kp*e;\nif ( (c >= 0) && (c < 100))\n{\n     I = I + (P*Dt)/Ti;\n}\nelse\n{\n  I = I;\n}\nc = P+I;\nif(c>100)\n{\n   c = 100;\n}\nif(c<0)\n{\n   c = 0;\n}\nPc = (c/100) * moc_grzalki;\nfor(m=0 ; m<NIS; m++)\n{\n float h = Dt/NIS;\n float G=F/V*(Twe-Twy)+Pc/(ro*cw*V);\nTwy=Twy+G*h;\n}"("F"=w371, "Twe"=w367, "V"=w372, "Twy"=w370, "Dt"=w365, "Twy_zad"="Twy [°C] zadane", "I"=w361, "c"=w360) -> ("Twy"=w368:dbl, "c"=w359:dbl, "e"=→"e uchyb":dbl, "I"=w362:dbl)
              "c [%] z regulatora" <- w359
              "I całkujacy" <- w362
            }
            frame "Dane wejściowe z pliku" {
              n131 = Divide(x=w378, y=100.0) -> (x/y=w388:dbl)
              n132 = Divide(x=w380, y=1000.0) -> (x/y=w383:dbl)
              n133 = Multiply(x=w388, y=12200.0) -> (x*y=w382:dbl)
              n134 = Divide(x=w376, y=60000.0) -> (x/y=w381:dbl)
              n135 = formula code="float T = V/F;\nfloat ro = 997.3;\nfloat cw = 4200;\n\nint NIS =1000;\n\nint m;\nfor(m=0 ; m<NIS; m++)\n{\n float h = Dt/NIS;\nfloat G=F/V*(Twe-Twy)+Pc/(ro*cw*V);\nTwy=Twy+G*h;\n}"("Pc"=w382, "F"=w381, "Twe"=w377, "V"=w383, "Twy"=w389, "Dt"=w375) -> ("Twy"=w379:dbl)
              "F [L/min] z pliku" <- w376
              "Twe [°C] z pliku" <- w377
              "c [%] Moc grzałki z pliku" <- w378
            }
          }
          "Twy [°C]" <- w335
          "Wykres Twy" <- w335
          n136 = Format Value(string ("")="", format string="%f", value (0)=w335) -> (output string=w333:string)
          n137 = Concatenate Strings(w333, "\r\n" ("string")) -> (w331:string)
          n138 = Write to Text File(file (use dialog)=w340, text=w331, error in=w339) -> (refnum out=w338:refnum<file>, error out=w337:errorcluster)  [unwired: 1 in, 1 out]
        }
        n139 = call <vilib>:"Add State(s) to Queue__JKI_lib_State_Machine.vi"("State(s) in Front (\"\")"="Simulation: UI_Stop" ("State(s) in Front (\"\")"), "State(s) in (\"\")"=w311) -> ("States Out"=w310:string)  [unwired: 13 in]
        n140 = Close File(refnum=w298, error in=w297) -> ()  [unwired: 2 out]
      }
      frame "New Category: 2" {
        # "Your code here.\n(You can make a copy of, or modify, this frame)"
        n141 = call <vilib>:"Add State(s) to Queue__JKI_lib_State_Machine.vi"("State(s) in (\"\")"=w393) -> ("States Out"=w392:string)  [unwired: 14 in]
      }
    }
  }
